vi "Find most recent folder.vi"(8 "error in (no error)":errorcluster, 10 "Directory to search":path, 11 "File path (used for pattern search)":path) -> (0 "error out":errorcluster, 3 "most recent folder":path)   [LabVIEW 2010, in "CAN Log Transfer and Convert.lvlib"]
uses:
  CAN Log Transfer and Convert.lvlib
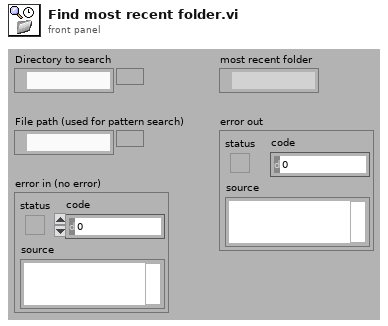
[diagram p1: front panel]
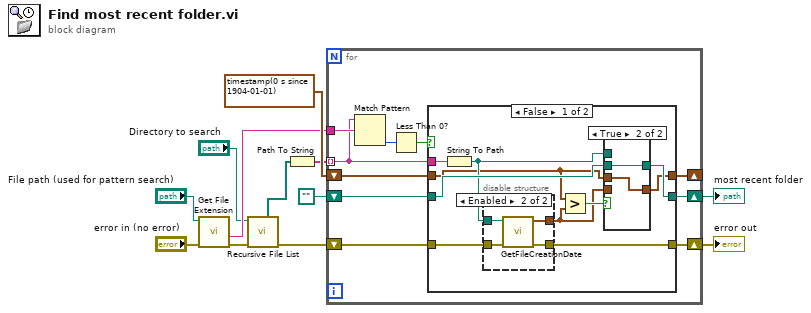
[diagram p0: block diagram]
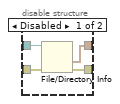
[diagram p2: hidden frame]
diagram:
  n1 = call <vilib>:"Get File Extension.vi"("error in (no error)"="error in (no error)", "file"="File path (used for pattern search)") -> ("error out"=w3:errorcluster, "filename without extension"=w4:string)  [unwired: 6 in, 2 out]
  n2 = call <vilib>:"Recursive File List.vi"("error in (no error)"=w3, "Folder Path"="Directory to search") -> ("error out"=w7:errorcluster, "All Folders"=w5:path[])  [unwired: 5 in, 3 out]
  n3 = Path To String(path=w5) -> (string=w6:string[])
  n4 = for {
    tunnel: w6 -> [w20] mode=indexing
    tunnel: w4 -> [w22]
    shift-right: [w17] -> w8
    shift-left: w7 -> [w18]
    shift-right: [w15] -> _
    shift-left: timestamp(0 s since 1904-01-01) ("last mod") -> [w16]
    shift-right: [w13] -> w11
    shift-left: path "" ("path") -> [w14]
    n5 = Match Pattern(string=w20, regular expression=w22) -> (offset past match=w21:i32)  [unwired: 1 in, 3 out]
    n6 = Less Than 0?(x=w21) -> (x < 0?=w19:bool)
    n7 = case shown="False" w19 {
      tunnel: w20 -> [w30 _]
      tunnel: w18 -> [w32 w45]
      tunnel: [w31 w45] -> w17
      tunnel: w16 -> [w25 w46]
      tunnel: [w23 w46] -> w15
      tunnel: w14 -> [w28 w47]
      tunnel: [w24 w47] -> w13
      frame False {
        n8 = String To Path(string=w30) -> (path=w27:path)
        n9 = disable-structure shown="Enabled" {
          disable-tunnel: w32 -> [w36 w38]
          disable-tunnel: [w35 w40] -> w31
          disable-tunnel: w27 -> [w34 w37]
          disable-tunnel: [w33 w39] -> w26
          frame Disabled {
            n10 = File/Directory Info(path=w34, error in=w36) -> (last mod=w33:timestamp, error out=w35:errorcluster)  [unwired: 5 out]
          }
          frame Enabled {
            n11 = call "GetFileCreationDate.vi"("error in (no error)"=w38, "File Path"=w37) -> ("error out"=w40:errorcluster, "File Created Date (UTC)"=w39:timestamp)  [unwired: 6 in]
          }
        }
        n12 = Greater?(x=w25, y=w26) -> (0:w29:bool)
        n13 = case shown="True" w29 {
          tunnel: w28 -> [_ w44]
          tunnel: [w42 w44] -> w24
          tunnel: w27 -> [w42 _]
          tunnel: [w41 w43] -> w23
          tunnel: w26 -> [w41 _]
          tunnel: w25 -> [_ w43]
          frame False {
          }
          frame True {
          }
        }
      }
      frame True {
      }
    }
  }
  "most recent folder" <- w11
  "error out" <- w8
